vi "{TMPL} MAIN - App.vi"() -> ()   [LabVIEW 2018, in "TLB` Template.lvlib" / "{TMPL} TLB`.lvclass"]
uses:
  {TMPL} TLB`.lvclass
  Application Components/Trigger API/System Trigger.ctl
  State Machine/State.ctl
  Core Components/Error Handler/TLB` Error Handler.lvclass
  Application Components/Configuration/{TMPL} Station Configuration.lvclass
  {TMPL} TLB`.lvclass/{TMPL} TLB`.ctl
  <vilib>/Utility/error.llb/Error Cluster From Error Code.vi
  <vilib>/ErrorRing/Error Ring.xnode
  Application Components/Trigger API/{TMPL} Trigger API.lvlib
  TLB` Template.lvlib
  Core Components/Actions/Actions.lvlib
  Core Components/Dependencies/TLB`_Dependencies.lvlib
panel:
  in  "Active Tab Selector":i32(listbox)
  in  "Connect Instrument":bool
  in  "Disconnect Instrument":bool
  in  "Initiate Analysis":bool
  in  "Stop Analysis":bool
  in  "Load Configuration":bool
  in  "Save Configuration":bool
  in  "Exit":bool
  in  "Main Tab":T1(tab)
  in  "VISA":refnum<visa-resource-name>
  out "error out":errorcluster
  in  "Preferences Button":bool
  out "Waveform Graph - Light":dbl[](graph)
  out "State":string
  out "Status":string
  # "TLB` Measurement Template"
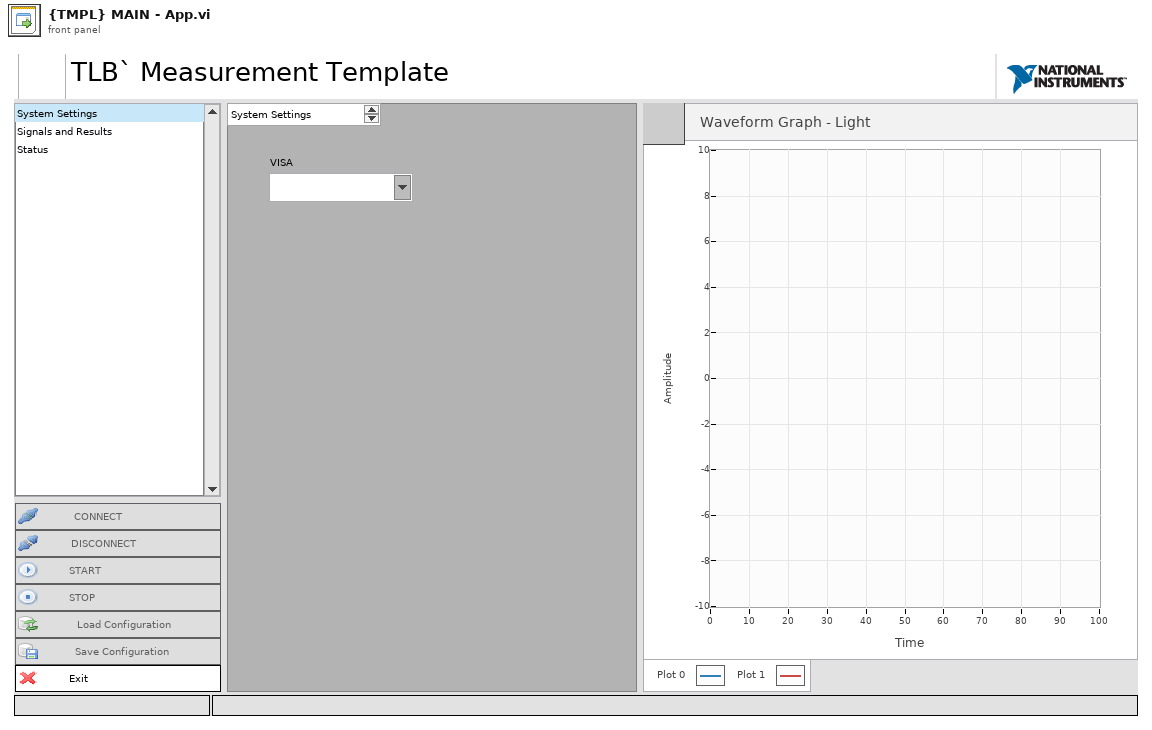
[diagram p1: front panel]
types:
  T1 = enum32{"System Settings", "Signals and Results", "Status"}
  T2 = typedef "TLB` Template.lvlib/{TMPL} TLB`.lvclass/State.ctl" = enum16{"<Startup>", "Idle", "Connected", "Monitoring", "Sweeping", "<Shutdown>", "<Error>"}
  T3 = enum16{"Close Display", "Clear References", "Close Error Handler"}
  T4 = enum16{"Clear SR", "Set Display", "Set Shifter", "Initialize Events", "Init Q"}
  T5 = typedef "TLB` Template.lvlib/{TMPL} Trigger API.lvlib/System Trigger.ctl" = enum16{"<None>", "Connect", "Start Acquisition", "Stop Acquisition", "Disconnect", "Load Configuration", "Save Configuration", "<Return to Safe State Actions>", "<Cache User Parameters>", "<Close Application>", "<Error>"}
  T6 = refnum<class "{TMPL} Station Configuration.lvclass">
  T7 = typedef "TLB` Template.lvlib/_UI CORE Event References.ctl" = cluster{"Exit Event":refnum<user-event>, "State Indicator":refnum<user-event>, "Status Indicator":refnum<user-event>}
  T8 = typedef "TLB` Template.lvlib/_UI APP Event References.ctl" = cluster{"Exit Event":refnum<user-event>}
  T9 = enum32{"Invalid", "Standard", "Closed", "Hidden", "Minimized", "Maximized"}
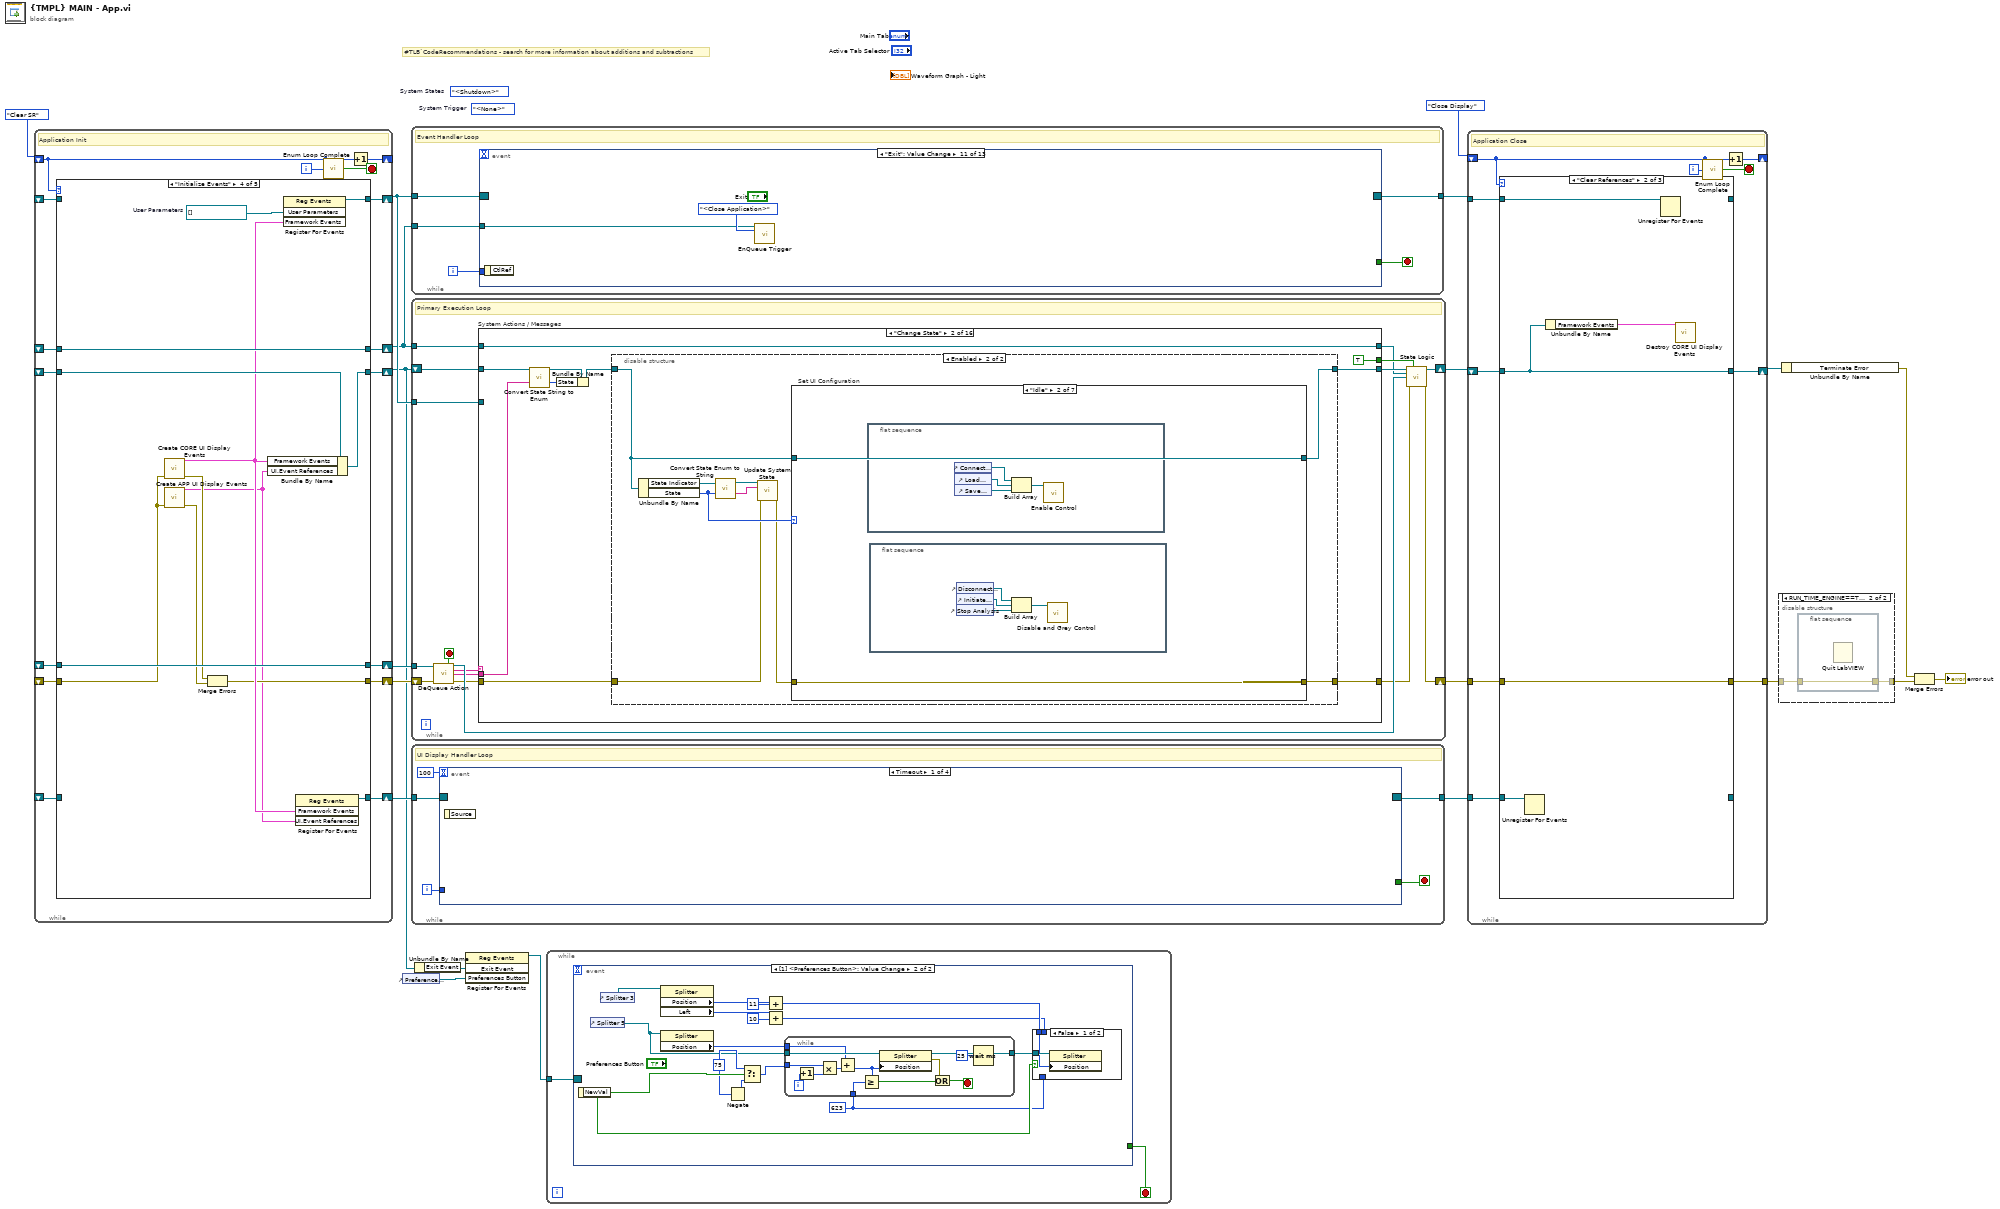
[diagram p0: block diagram]
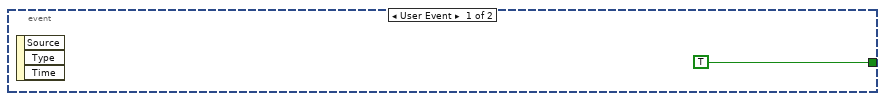
[diagram p2: hidden frame]
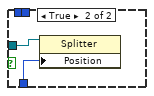
[diagram p3: hidden frame]
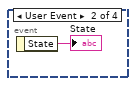
[diagram p4: hidden frame]
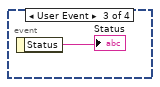
[diagram p5: hidden frame]
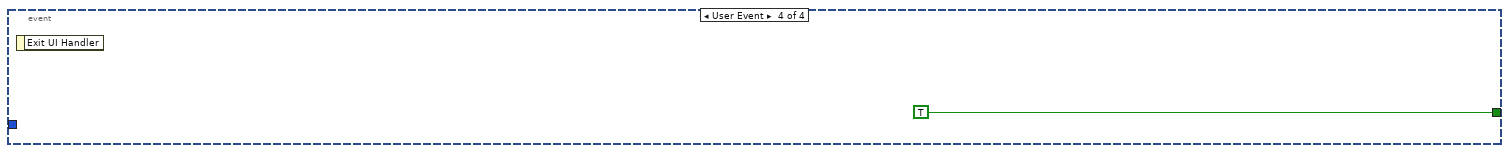
[diagram p6: hidden frame]
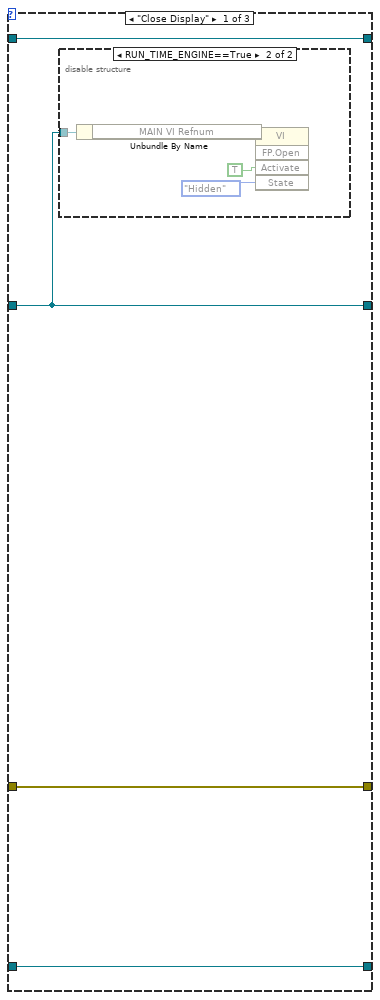
[diagram p8: hidden frame]
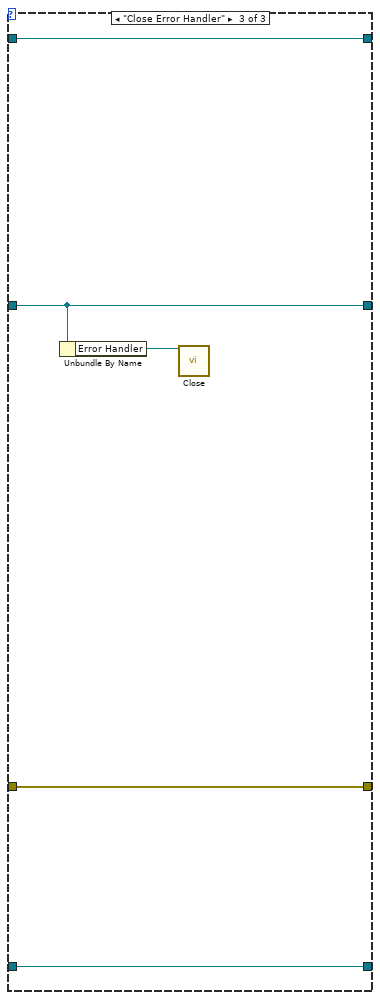
[diagram p10: hidden frame]
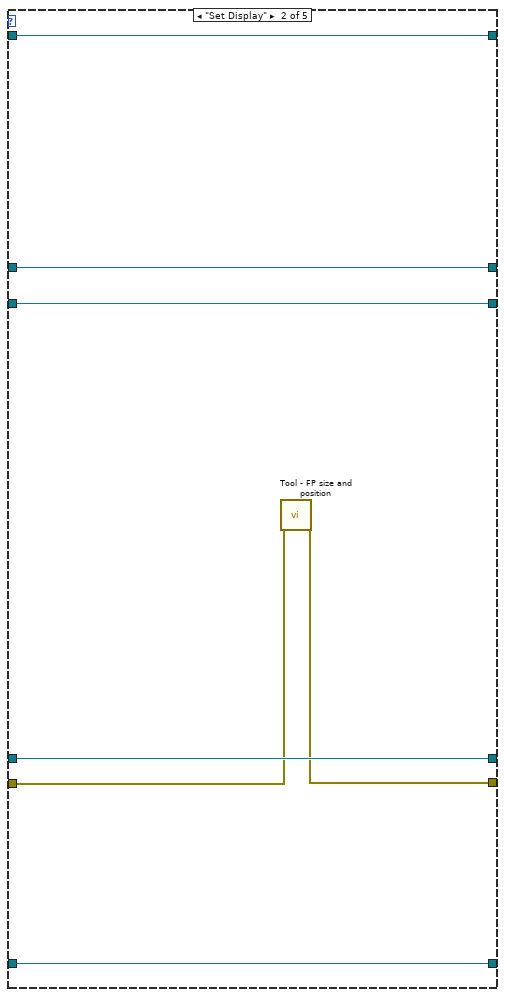
[diagram p12: hidden frame]
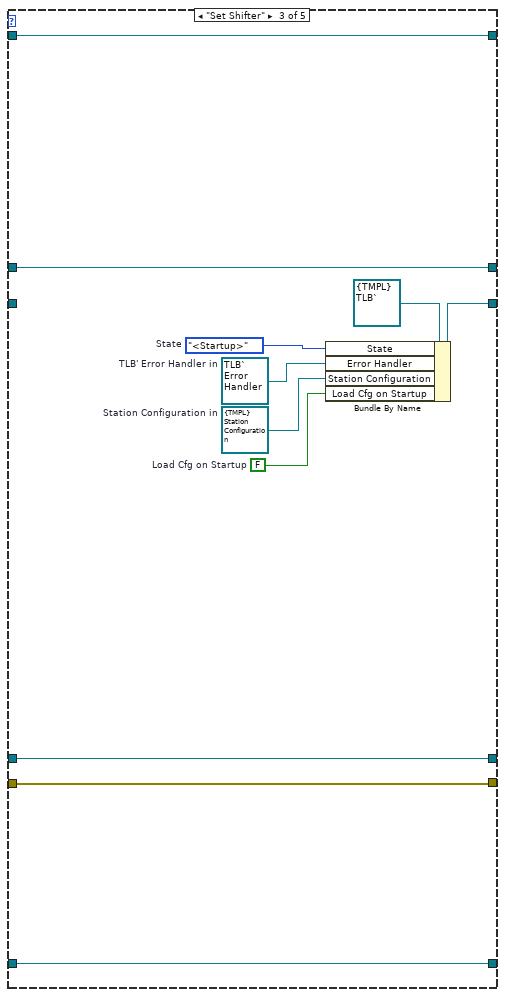
[diagram p13: hidden frame]
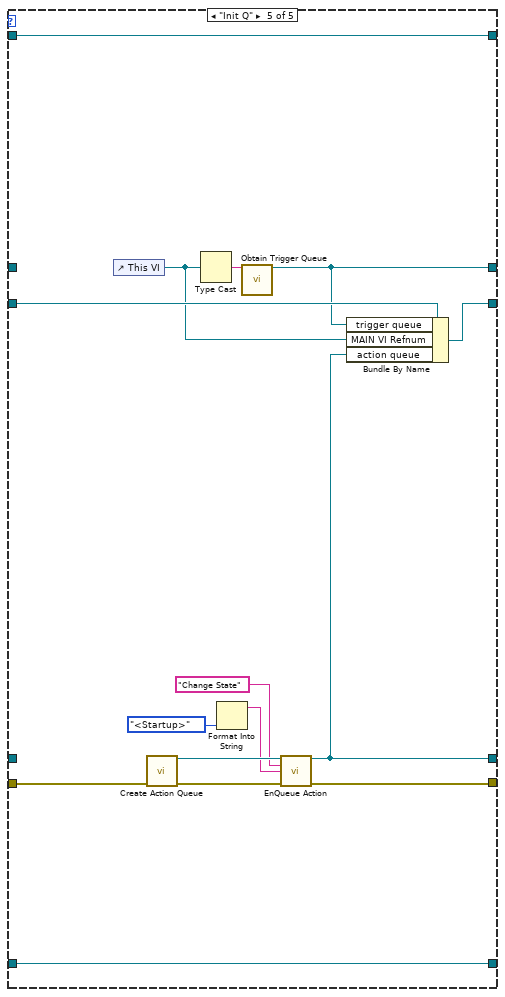
[diagram p14: hidden frame]
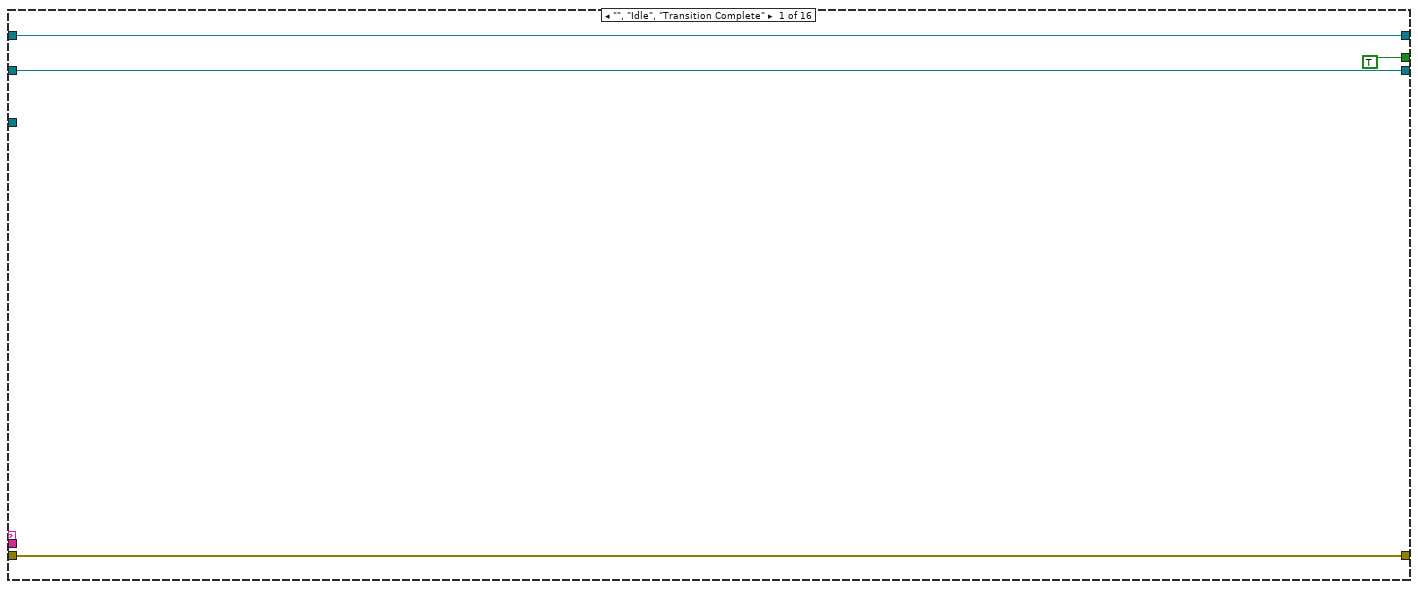
[diagram p15: hidden frame]
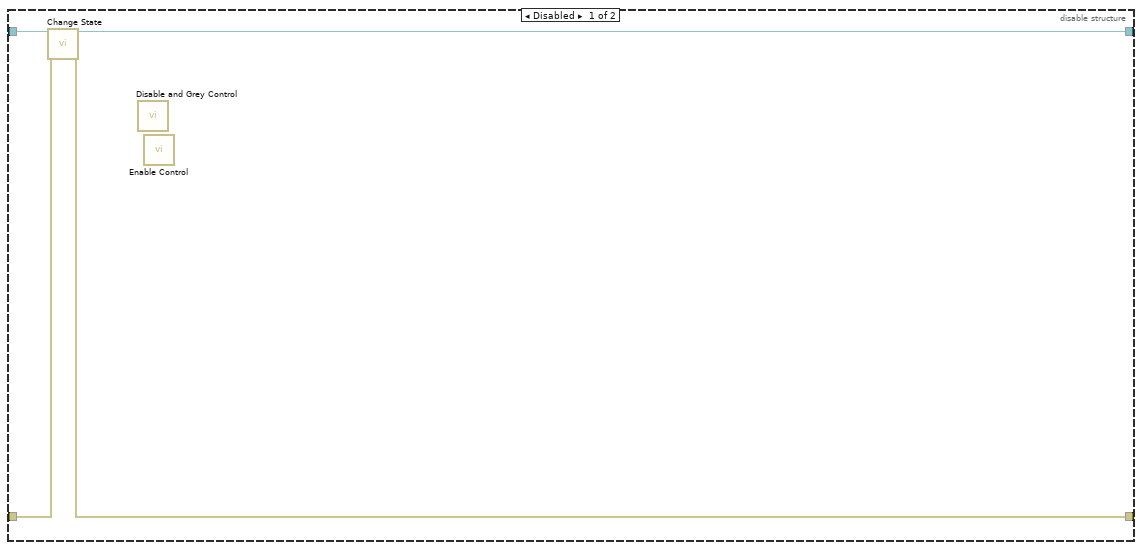
[diagram p16: hidden frame]
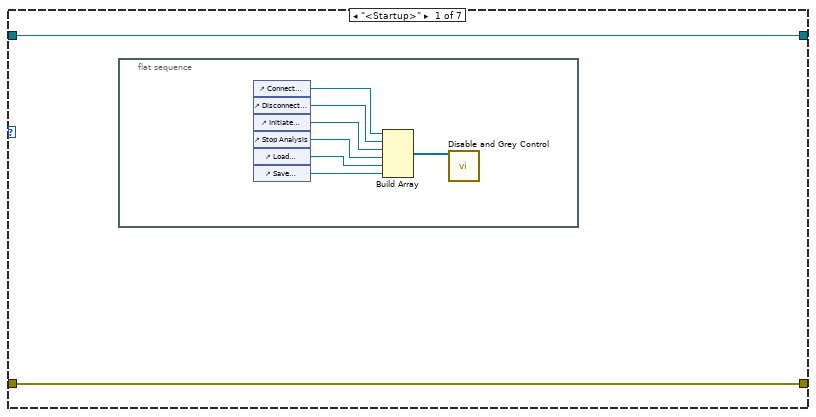
[diagram p17: hidden frame]
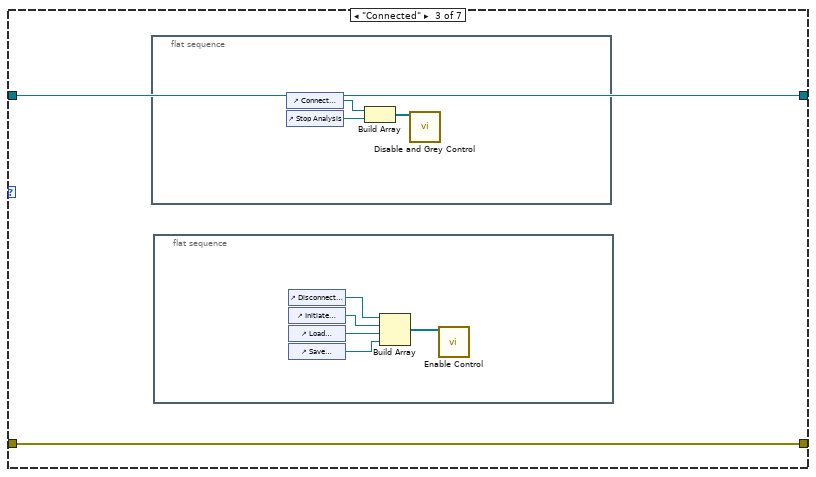
[diagram p18: hidden frame]
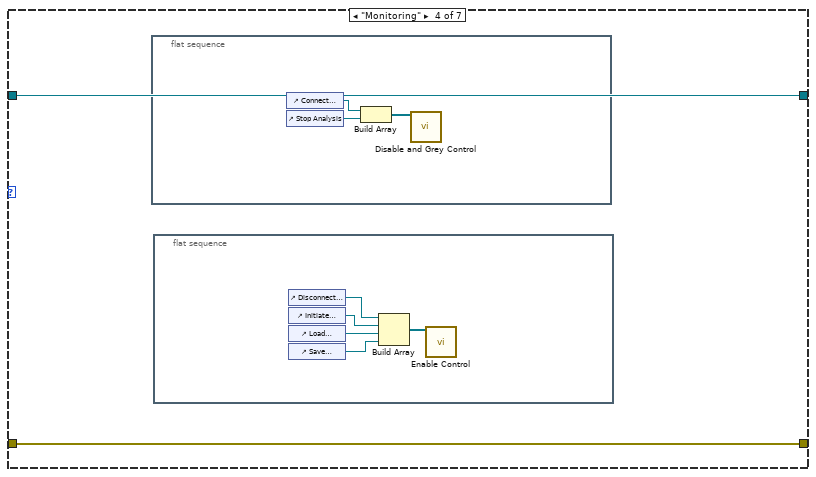
[diagram p19: hidden frame]
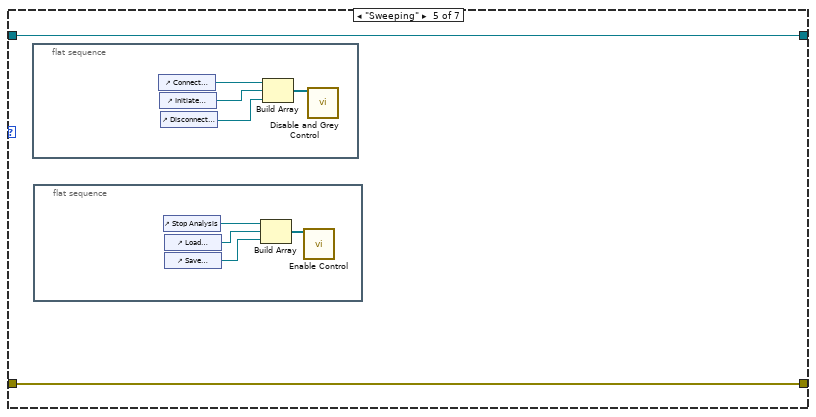
[diagram p20: hidden frame]
diagram:
  (unwired) State."<Shutdown>"  # System States
  (unwired) System_Trigger."<None>"  # System Trigger
  # "#TLB`CodeRecommendations - search for more information about additions and subtractions"
  n1 = while {
    shift-right: [w32] -> _
    shift-left: T4."Clear SR" -> [w21]
    shift-right: [w36] -> w20
    shift-left: _ -> [w31]
    shift-right: [w33] -> w15
    shift-left: _ -> [w30]
    shift-right: [w35] -> w14
    shift-left: _ -> [w29]
    shift-right: [w34] -> w4
    shift-left: _ -> [w28]
    shift-right: [w27] -> w10
    shift-left: _ -> [w26]
    shift-right: [w25] -> w13
    shift-left: _ -> [w24]
    i -> [w22]
    stop <- w23 stop-if-true
    # "Application Init"
    n2 = case shown="\"Initialize Events\"" w21 {
      tunnel: [_ w41 w54 w67 w68] -> w36
      tunnel: [_ w39 w53 w57 w74] -> w33
      tunnel: [_ w43 w49 w65 w80] -> w34
      tunnel: [_ w42 w52 w64 w82] -> w35
      tunnel: w31 -> [_ w41 w54 w67 _]
      tunnel: w30 -> [_ w40 w53 w56 w76]
      tunnel: w29 -> [_ w42 w52 _ w82]
      tunnel: w28 -> [_ w43 _ w66 w81]
      tunnel: [_ w38 w51 w63 w69] -> w27
      tunnel: w26 -> [_ w38 w51 w63 _]
      tunnel: [_ w37 w47 w61 w77] -> w25
      tunnel: w24 -> [_ w37 w47 _ w77]
      frame "Clear SR" {
      }
      frame "Set Display" {
        n3 = call "Tool - FP size and position.vi"("error in (no error)"=w40) -> ("error out"=w39:errorcluster)  [unwired: 17 in, 1 out]
      }
      frame "Set Shifter" {
        w44 = FALSE  # Load Cfg on Startup
        w45 = T6 refnum  # Station Configuration in
        w46 = refnum<class "TLB` Error Handler.lvclass"> refnum  # TLB' Error Handler in
        w50 = State."<Startup>"  # State
        n4 = Bundle By Name(cluster=refnum<class "{TMPL} TLB`.lvclass"> refnum ("TLB` Template.lvlib:TLB' Template.lvclass"), "State"=w50, "Error Handler"=w46, "Station Configuration"=w45, "Load Cfg on Startup"=w44) -> (w49:refnum<class "{TMPL} TLB`.lvclass">)
      }
      frame "Initialize Events" {
        w62 = refnum<vi>[] []  # User Parameters
        n5 = call "Create CORE UI Display Events.vi"("error in"=w56) -> ("Framework Events"=w60:T7, "error out"=w59:errorcluster)  [unwired: 13 in]
        n6 = call "Create APP UI Display Events.vi"("error in"=w56) -> ("UI.Event References"=w55:T8, "error out"=w58:errorcluster)  [unwired: 13 in]
        n7 = Merge Errors(w59, w58) -> (w57:errorcluster)
        n8 = Bundle By Name(cluster=w66, "Framework Events"=w60, "UI.Event References"=w55) -> (w65:refnum<class "{TMPL} TLB`.lvclass">)
        n9 = register-events(w62, w60) -> (reference out=w64:refnum<event-registration>)  [unwired: 2 in, 1 out]
        n10 = register-events(w60, w55) -> (reference out=w61:refnum<event-registration>)  [unwired: 2 in, 1 out]
      }
      frame "Init Q" {
        n11 = control-ref of="This VI"() -> (w79:refnum<vi>)
        n12 = call "Create Action Queue.vi"("error in"=w76) -> ("action queue out"=w73:refnum<queue>, "error out"=w75:errorcluster)  [unwired: 13 in]
        n13 = Type Cast(x=w79) -> (*(type *) &x=w70:string)  [unwired: 1 in]
        n14 = Format Into String(State."<Startup>" ("State")) -> (resulting string=w71:string)  [unwired: 3 in, 1 out]
        n15 = call "Obtain Trigger Queue.vi"("trigger queue name"=w70) -> ("trigger queue out"=w69:refnum<queue>)  [unwired: 13 in, 1 out]
        n16 = call "EnQueue Action.vi"("action queue in"=w73, "action"="Change State" ("Message Name"), "data in"=w71, "error in"=w75) -> ("action queue out"=w68:refnum<queue>, "error out"=w74:errorcluster)  [unwired: 10 in]
        n17 = Bundle By Name(cluster=w81, "trigger queue"=w69, "MAIN VI Refnum"=w79, "action queue"=w68) -> (w80:refnum<class "{TMPL} TLB`.lvclass">)
      }
    }
    n18 = call "Enum Loop Complete.vi"("Current State Enum"=w21, "Itteration"=w22) -> ("Loop Complete?"=w23:bool)  [unwired: 12 in, 1 out]
    n19 = Increment(x=w21) -> (x+1=w32:T4)
  }
  n20 = control-ref of="Preferences Button"() -> (w1:refnum<vi>)
  n21 = while {
    shift-right: [w93] -> w12
    shift-left: w15 -> [w88]
    shift-right: [w95] -> w16
    shift-left: w4 -> [w97]
    tunnel: w20 -> [w89]
    tunnel: w14 -> [w96]
    tunnel: w10 -> [w92]
    stop <- w87 stop-if-true
    # "Primary Execution Loop"
    n22 = call "DeQueue Action.vi"("action queue in"=w89, "error in"=w88) -> ("exit?"=w87:bool, "action queue out"=w98:refnum<queue>, "action"=w85:string, "action value"=w83:string, "error out"=w86:errorcluster)  [unwired: 8 in, 1 out]
    n23 = case "System Actions / Messages" shown="\"Change State\"" w85 {
      selector: w85 -> [_ _ _ _ _ _ _ _ _ _ _ _ _ _ _ w275]
      tunnel: [w102 w109 w190 w194 w195 w204 w213 w229 w238 w244 w247 w252 w257 w258 w270 w274] -> w90
      tunnel: w86 -> [w102 w108 w190 w194 w195 w207 w213 w229 w236 w244 w247 w251 w257 w259 w271 _]
      tunnel: w97 -> [w99 w107 w187 w193 w198 w205 w216 w228 w232 w243 w246 w254 w256 w262 w273 w277]
      tunnel: [w99 w103 w191 w193 w197 w210 w219 w228 w233 w243 w246 w254 w256 w261 w272 w277] -> w94
      tunnel: w96 -> [_ _ _ _ _ _ w217 _ _ _ _ _ _ _ _ _]
      tunnel: [w100 w110 w189 w192 w199 w211 w218 w227 w241 w242 w245 w249 w255 w265 w266 w276] -> w84
      tunnel: w92 -> [w100 w110 w189 w192 w199 w211 w218 w227 w241 w242 w245 w249 w255 w265 w266 w276]
      tunnel: [TRUE TRUE _ _ _ _ _ _ _ _ _ _ _ _ _ _] -> w91
      tunnel: w83 -> [_ w106 _ _ _ _ _ _ _ _ _ _ _ _ _ _]
      frame "", "Idle", "Transition Complete" {
      }
      frame "Change State" {
        n24 = call "Convert State String to Enum.vi"("state in"=w106) -> ("state out"=w105:T2)  [unwired: 13 in, 1 out]
        n25 = Bundle By Name(cluster=w107, "State"=w105) -> (w104:refnum<class "{TMPL} TLB`.lvclass">)
        n26 = disable-structure shown="Enabled" {
          disable-tunnel: [w115 w116] -> w109
          disable-tunnel: w108 -> [w114 w117]
          disable-tunnel: w104 -> [w113 w119]
          disable-tunnel: [w112 w118] -> w103
          frame Disabled {
            n27 = call "Change State.vi"("TLB' data in"=w113, "error in"=w114) -> ("TLB' data out"=w112:refnum<class "{TMPL} TLB`.lvclass">, "error out"=w115:errorcluster)  [unwired: 12 in]
            n28 = call "Disable and Grey Control.vi"() -> ()  [unwired: 15 in, 1 out]
            n29 = call "Enable Control.vi"() -> ()  [unwired: 15 in, 1 out]
          }
          frame Enabled {
            n30 = Unbundle By Name(w119) -> ("State Indicator"=w120:refnum<user-event>, "State"=w123:T2)
            n31 = call "Convert State Enum to String.vi"("state in"=w123) -> ("state out"=w121:string)  [unwired: 13 in, 1 out]
            n32 = call "Update System State.vi"("State Indicator"=w120, "system state message"=w121, "error in"=w117) -> ("error out"=w122:errorcluster)  [unwired: 12 in]
            n33 = case "Set UI Configuration" shown="\"Idle\"" w123 {
              tunnel: [w124 w134 w144 w154 w164 w176 w184] -> w116
              tunnel: w122 -> [w124 w134 w144 w154 w164 w176 w184]
              tunnel: [w125 w133 w143 w153 w163 w175 w185] -> w118
              tunnel: w119 -> [w125 w133 w143 w153 w163 w175 w185]
              frame "<Startup>" {
                n34 = flat-sequence {
                  frame #0 {
                    n35 = control-ref of="Connect Instrument"() -> (w132:refnum<vi>)
                    n36 = control-ref of="Disconnect Instrument"() -> (w131:refnum<vi>)
                    n37 = control-ref of="Initiate Analysis"() -> (w130:refnum<vi>)
                    n38 = control-ref of="Stop Analysis"() -> (w129:refnum<vi>)
                    n39 = control-ref of="Load Configuration"() -> (w128:refnum<vi>)
                    n40 = control-ref of="Save Configuration"() -> (w127:refnum<vi>)
                    n41 = Build Array(w132, w131, w130, w129, w128, w127) -> (w126:refnum<vi>[])
                    n42 = call "Disable and Grey Control.vi"("Control Ref"=w126) -> ()  [unwired: 14 in, 1 out]
                  }
                }
              }
              frame "Idle" {
                n43 = flat-sequence {
                  frame #0 {
                    n44 = control-ref of="Connect Instrument"() -> (w140:refnum<vi>)
                    n45 = control-ref of="Load Configuration"() -> (w142:refnum<vi>)
                    n46 = control-ref of="Save Configuration"() -> (w141:refnum<vi>)
                    n47 = Build Array(w140, w142, w141) -> (w139:refnum<vi>[])
                    n48 = call "Enable Control.vi"("Control Ref"=w139) -> ()  [unwired: 14 in, 1 out]
                  }
                }
                n49 = flat-sequence {
                  frame #0 {
                    n50 = control-ref of="Disconnect Instrument"() -> (w138:refnum<vi>)
                    n51 = control-ref of="Initiate Analysis"() -> (w137:refnum<vi>)
                    n52 = control-ref of="Stop Analysis"() -> (w136:refnum<vi>)
                    n53 = Build Array(w138, w137, w136) -> (w135:refnum<vi>[])
                    n54 = call "Disable and Grey Control.vi"("Control Ref"=w135) -> ()  [unwired: 14 in, 1 out]
                  }
                }
              }
              frame "Connected" {
                n55 = flat-sequence {
                  frame #0 {
                    n56 = control-ref of="Connect Instrument"() -> (w152:refnum<vi>)
                    n57 = control-ref of="Stop Analysis"() -> (w151:refnum<vi>)
                    n58 = Build Array(w152, w151) -> (w150:refnum<vi>[])
                    n59 = call "Disable and Grey Control.vi"("Control Ref"=w150) -> ()  [unwired: 14 in, 1 out]
                  }
                }
                n60 = flat-sequence {
                  frame #0 {
                    n61 = control-ref of="Disconnect Instrument"() -> (w149:refnum<vi>)
                    n62 = control-ref of="Initiate Analysis"() -> (w148:refnum<vi>)
                    n63 = control-ref of="Load Configuration"() -> (w147:refnum<vi>)
                    n64 = control-ref of="Save Configuration"() -> (w146:refnum<vi>)
                    n65 = Build Array(w149, w148, w147, w146) -> (w145:refnum<vi>[])
                    n66 = call "Enable Control.vi"("Control Ref"=w145) -> ()  [unwired: 14 in, 1 out]
                  }
                }
              }
              frame "Monitoring" {
                n67 = flat-sequence {
                  frame #0 {
                    n68 = control-ref of="Connect Instrument"() -> (w162:refnum<vi>)
                    n69 = control-ref of="Stop Analysis"() -> (w161:refnum<vi>)
                    n70 = Build Array(w162, w161) -> (w160:refnum<vi>[])
                    n71 = call "Disable and Grey Control.vi"("Control Ref"=w160) -> ()  [unwired: 14 in, 1 out]
                  }
                }
                n72 = flat-sequence {
                  frame #0 {
                    n73 = control-ref of="Disconnect Instrument"() -> (w159:refnum<vi>)
                    n74 = control-ref of="Initiate Analysis"() -> (w158:refnum<vi>)
                    n75 = control-ref of="Load Configuration"() -> (w157:refnum<vi>)
                    n76 = control-ref of="Save Configuration"() -> (w156:refnum<vi>)
                    n77 = Build Array(w159, w158, w157, w156) -> (w155:refnum<vi>[])
                    n78 = call "Enable Control.vi"("Control Ref"=w155) -> ()  [unwired: 14 in, 1 out]
                  }
                }
              }
              frame "Sweeping" {
                n79 = flat-sequence {
                  frame #0 {
                    n80 = control-ref of="Connect Instrument"() -> (w172:refnum<vi>)
                    n81 = control-ref of="Initiate Analysis"() -> (w170:refnum<vi>)
                    n82 = control-ref of="Disconnect Instrument"() -> (w169:refnum<vi>)
                    n83 = Build Array(w172, w170, w169) -> (w171:refnum<vi>[])
                    n84 = call "Disable and Grey Control.vi"("Control Ref"=w171) -> ()  [unwired: 14 in, 1 out]
                  }
                }
                n85 = flat-sequence {
                  frame #0 {
                    n86 = control-ref of="Stop Analysis"() -> (w166:refnum<vi>)
                    n87 = control-ref of="Load Configuration"() -> (w168:refnum<vi>)
                    n88 = control-ref of="Save Configuration"() -> (w167:refnum<vi>)
                    n89 = Build Array(w166, w168, w167) -> (w165:refnum<vi>[])
                    n90 = call "Enable Control.vi"("Control Ref"=w165) -> ()  [unwired: 14 in, 1 out]
                  }
                }
              }
              frame "<Shutdown>" {
                n91 = flat-sequence {
                  frame #0 {
                    n92 = control-ref of="Connect Instrument"() -> (w183:refnum<vi>)
                    n93 = control-ref of="Disconnect Instrument"() -> (w182:refnum<vi>)
                    n94 = control-ref of="Initiate Analysis"() -> (w181:refnum<vi>)
                    n95 = control-ref of="Stop Analysis"() -> (w180:refnum<vi>)
                    n96 = control-ref of="Load Configuration"() -> (w179:refnum<vi>)
                    n97 = control-ref of="Save Configuration"() -> (w178:refnum<vi>)
                    n98 = Build Array(w183, w182, w181, w180, w179, w178) -> (w177:refnum<vi>[])
                    n99 = call "Disable and Grey Control.vi"("Control Ref"=w177) -> ()  [unwired: 14 in, 1 out]
                  }
                }
                n100 = control-ref of="Preferences Button"() -> (w174:refnum<vi>)
                n101 = property class="Bool (strict)"(reference=w174, "Val(Sgnl)"=TRUE ("Value (Signaling)")) -> ()  [unwired: 1 in, 2 out]
              }
              frame "<Error>" {
              }
            }
          }
        }
      }
      frame "Cache User Parameters" {
        n102 = Bundle By Name(cluster=w187, "Active Item Tag"="" ("User Data.Active Item Tag"), "VISA"="VISA") -> (w191:refnum<class "{TMPL} TLB`.lvclass">)
      }
      frame "/*********INITialize********/" {
      }
      frame "INIT::Load Application Base Path" {
        n103 = disable-structure shown="Default" {
          disable-tunnel: [w200 w202] -> w196
          frame condition #0 (active) {
            n104 = Current VI's Path() -> (path=w201:path)
            n105 = Strip Path(path=w201) -> (stripped path=w200:path)  [unwired: 1 out]
          }
          frame condition #1 {
            n106 = call <vilib>:"Application Directory.vi"() -> ("Application Directory"=w202:path)
          }
        }
        n107 = Bundle By Name(cluster=w198, "Application Base Path"=w196) -> (w197:refnum<class "{TMPL} TLB`.lvclass">)
      }
      frame "INIT::Initialize Error Handler" {
        n108 = Unbundle By Name(w205) -> ("Application Base Path"=w212:path)
        n109 = Unbundle By Name(w205) -> ("Error Handler"=w206:refnum<class "TLB` Error Handler.lvclass">)
        n110 = Build Path(base path=w212, name or relative path="System Level Errors\\System Errors.txt") -> (appended path=w208:path)
        n111 = call-dynamic "Open.vi"("error handler in"=w206, "error log path in"=w208, "error in"=w207) -> ("error handler out"=w209:refnum<class "TLB` Error Handler.lvclass">, "error out"=w204:errorcluster)  [unwired: 11 in]
        n112 = Bundle By Name(cluster=w205, "Error Handler"=w209) -> (w210:refnum<class "{TMPL} TLB`.lvclass">)
      }
      frame "INIT::Register User Parameters" {
        n113 = disable-structure shown="Enabled" {
          disable-tunnel: [w220 refnum<vi>[] [] ("User Parameter Controls")] -> w215
          frame Enabled {
            n114 = stacked-sequence "Stacked Sequence Structure :: Allows for a lot of controls" {
              tunnel: [w222] -> w220
              frame #0 {
                n115 = control-ref of="VISA"() -> (w221:refnum<vi>)
                n116 = Build Array(w221) -> (w222:refnum<vi>[])
              }
            }
          }
          frame Disabled {
          }
        }
        n117 = Build Array (concatenate)(w215) -> (w214:refnum<vi>[])
        n118 = register-events(reference=w217, w214) -> ()  [unwired: 2 in, 2 out]
        n119 = Bundle By Name(cluster=w216, "User Parameter Controls"=w214) -> (w219:refnum<class "{TMPL} TLB`.lvclass">)
      }
      frame "INIT::FP Values" {
        w224 = 0
        # "#TLB`CodeRecommendations - initialize FP values here"
        n120 = property on="Main Tab" class="TabCtl (strict)"() -> ("Pages"=w226:refnum<vi>[])  [unwired: 2 in, 2 out]
        n121 = for {
          tunnel: w226 -> [w231] mode=indexing
          tunnel: [w230] -> w225 mode=indexing
          n122 = property class="Page"(reference=w231) -> ("TabCaption"=w230:string)  [unwired: 1 in, 2 out]
        }
        n123 = local write "Active Tab Selector"(w224) -> ()
        n124 = local write "Main Tab"(w224) -> ()
        n125 = property on="Active Tab Selector" class="LstBox (strict)"("Item Names"=w225) -> ()  [unwired: 2 in, 2 out]
      }
      frame "CFG::Load Station Configuration" {
        n126 = Unbundle By Name(w232) -> ("Application Base Path"=w240:path)
        n127 = Unbundle By Name(w232) -> ("Station Configuration"=w235:T6)
        n128 = Build Path(base path=w240, name or relative path="System Configuration\\Station Configuration.ini") -> (appended path=w237:path)
        n129 = call-dynamic "Load Configuration.vi"("INI Station Configuration in"=w235, "INI file path in"=w237, "error in"=w236) -> ("INI Station Configuration out"=w234:T6, "error out"=w238:errorcluster)  [unwired: 11 in]
        n130 = Bundle By Name(cluster=w232, "Station Configuration"=w234) -> (w233:refnum<class "{TMPL} TLB`.lvclass">)
      }
      frame "/*********PRImary EXEcution********/" {
      }
      frame "/*********SHUTDOWN********/" {
      }
      frame "Exit" {
        w250 = refnum<class> refnum  # event data
        # "Don't wire 'Error In'\nMust Execute Regardless"
        n131 = Unbundle By Name(w254) -> ("Exit Event"=w248:refnum<user-event>)
        n132 = Generate User Event(user event=w248, event data cluster=w250) -> (error out=w253:errorcluster)  [unwired: 2 in, 1 out]
        n133 = Merge Errors(w251, w253) -> (w252:errorcluster)
      }
      frame "/*********ERRor Handler********/" {
      }
      frame "ERR::Log" {
        n134 = Unbundle By Name(w262) -> ("Error Handler"=w264:refnum<class "TLB` Error Handler.lvclass">)
        n135 = call-dynamic "Log.vi"("error handler in"=w264) -> ("error handler out"=w263:refnum<class "TLB` Error Handler.lvclass">, "error out"=w260:errorcluster)  [unwired: 13 in]
        n136 = Bundle By Name(cluster=w262, "Error Handler"=w263) -> (w261:refnum<class "{TMPL} TLB`.lvclass">)
        n137 = Merge Errors(w259, w260) -> (w258:errorcluster)
      }
      frame "ERR::Dialog" {
        n138 = Unbundle By Name(w273) -> ("Error Handler"=w269:refnum<class "TLB` Error Handler.lvclass">)
        n139 = call-dynamic "Dialog.vi"("error handler in"=w269, "trigger queue in"=w266) -> ("error handler out"=w268:refnum<class "TLB` Error Handler.lvclass">, "error out"=w267:errorcluster)  [unwired: 12 in]
        n140 = Merge Errors(w271, w267) -> (w270:errorcluster)
        n141 = Bundle By Name(cluster=w273, "Error Handler"=w268) -> (w272:refnum<class "{TMPL} TLB`.lvclass">)
      }
      frame Default {
        n142 = xnode "Error Ring"("parameter 0"=w275) -> ("error out"=w274:errorcluster)
      }
    }
    n143 = call "State Logic.vi"("TLB' data in"=w94, "process state logic enable"=w91, "trigger queue in"=w84, "action queue in"=w98, "error in"=w90) -> ("TLB' data out"=w95:refnum<class "{TMPL} TLB`.lvclass">, "error out"=w93:errorcluster)  [unwired: 9 in]
  }
  n144 = while {
    tunnel: w13 -> [w289]
    tunnel: [w285] -> w11
    i -> [w288]
    stop <- w287 stop-if-true
    # "UI Display Handler Loop"
    n145 = event shown="[0] Timeout" {
      selector: w289 -> [_ _ _ _]
      dyn-events: [_ _ _ _] -> w285
      timeout: 100 -> [_ _ _ _]
      tunnel: w288 -> [_ _ _ _]
      tunnel: [_ _ _ TRUE] -> w287
      event Timeout {
        n146 = event-data() -> ()  [unwired: 2 out]
      }
      event User Event {
        n147 = event-data() -> ("State"=→"State":string)  [unwired: 1 out]
      }
      event User Event {
        n148 = event-data() -> ("Status"=→"Status":string)  [unwired: 1 out]
      }
      event User Event {
        n149 = event-data() -> ()  [unwired: 2 out]
      }
    }
  }
  n150 = while {
    tunnel: w14 -> [w296]
    tunnel: [w295] -> w17
    tunnel: w10 -> [w293]
    i -> [w294]
    stop <- w297 stop-if-true
    # "Event Handler Loop"
    n151 = event shown="[10] \"Exit\": Value Change" {
      selector: w296 -> [_ _ _ _ _ _ _ _ _ _ _ _ _]
      dyn-events: [_ _ _ _ _ _ _ _ _ _ _ _ _] -> w295
      timeout: _ -> [_ _ _ _ _ _ _ _ _ _ _ _ _]
      tunnel: [_ _ TRUE ("NewVal") _ _ _ _ _ _ _ _ _ _] -> w297
      tunnel: w294 -> [_ _ _ _ _ _ _ _ _ _ _ _ _]
      tunnel: w293 -> [w298 _ w310 w314 w317 w319 w321 w323 w325 w327 w328 _ _]
      event Panel Close? {
        w300 = TRUE  # Discard?
        n152 = event-data() -> ()  [unwired: 2 out]
        n153 = call "EnQueue Trigger.vi"("trigger queue in"=w298, "system trigger"=System_Trigger."<Close Application>" ("System Trigger")) -> ()  [unwired: 12 in, 2 out]
        n154 = event-data("Discard?"=w300) -> ()  [unwired: 1 in, 1 out]
      }
      event Mouse Down {
        n155 = event-data() -> ("Button"=w301:u16, "Mods.Double Click"=w302:bool)  [unwired: 1 out]
        n156 = Equal?(x=u16 2, y=w301) -> (x = y?=w304:bool)
        n157 = Compound Arithmetic op=AND(w304, w302) -> (w303:bool)
        n158 = case "Toggle Menu Visibility :: double RIGHT click on logo" shown="True" w303 {
          frame False {
          }
          frame True {
            n159 = property class="VI"() -> (reference out=w308:refnum<vi>, "TB.Visible"=w307:bool)  [unwired: 2 in, 1 out]
            n160 = Not(x=w307) -> (.not. x?=w306:bool)
            n161 = property class="VI"(reference=w308, "TB.Visible"=w306, "Front Panel.ShowMenuBar"=w306) -> ()  [unwired: 1 in, 2 out]
          }
        }
      }
      event User Event {
        n162 = event-data() -> ()  [unwired: 2 out]
        n163 = call "EnQueue Trigger.vi"("trigger queue in"=w310, "system trigger"=System_Trigger."<Close Application>" ("System Trigger")) -> ()  [unwired: 12 in, 2 out]
      }
      event Value Change {
        n164 = event-data() -> ()  [unwired: 2 out]
        n165 = call "EnQueue Trigger.vi"("trigger queue in"=w314, "system trigger"=System_Trigger."<Cache User Parameters>" ("System Trigger")) -> ("trigger queue out"=w313:refnum<queue>)  [unwired: 12 in, 1 out]
        n166 = event "use this event case to register a SPEICIFIC 'User Parameter' for a SPECIFIC action" shown="[0] Timeout" {
          selector: _ -> [_]
          dyn-events: _ -> [_]
          timeout: 0 -> [_]
          tunnel: w313 -> [_]
          event Timeout {
            n167 = event-data() -> ()  [unwired: 1 in, 1 out]
          }
        }
      }
      event "Connect Instrument": Value Change {
        n168 = event-data() -> ()  [unwired: 2 out]
        n169 = call "EnQueue Trigger.vi"("trigger queue in"=w317, "system trigger"=System_Trigger."Connect" ("System Trigger")) -> ()  [unwired: 12 in, 2 out]
      }
      event "Disconnect Instrument": Value Change {
        n170 = event-data() -> ()  [unwired: 2 out]
        n171 = call "EnQueue Trigger.vi"("trigger queue in"=w319, "system trigger"=System_Trigger."Disconnect" ("System Trigger")) -> ()  [unwired: 12 in, 2 out]
      }
      event "Initiate Analysis": Value Change {
        n172 = event-data() -> ()  [unwired: 2 out]
        n173 = call "EnQueue Trigger.vi"("trigger queue in"=w321, "system trigger"=System_Trigger."Start Acquisition" ("System Trigger")) -> ()  [unwired: 12 in, 2 out]
      }
      event "Stop Analysis": Value Change {
        n174 = event-data() -> ()  [unwired: 2 out]
        n175 = call "EnQueue Trigger.vi"("trigger queue in"=w323, "system trigger"=System_Trigger."Stop Acquisition" ("System Trigger")) -> ()  [unwired: 12 in, 2 out]
      }
      event "Save Configuration": Value Change {
        n176 = event-data() -> ()  [unwired: 2 out]
        n177 = call "EnQueue Trigger.vi"("trigger queue in"=w325, "system trigger"=System_Trigger."Save Configuration" ("System Trigger")) -> ()  [unwired: 12 in, 2 out]
      }
      event "Load Configuration": Value Change {
        n178 = event-data() -> ()  [unwired: 2 out]
        n179 = call "EnQueue Trigger.vi"("trigger queue in"=w327, "system trigger"=System_Trigger."Load Configuration" ("System Trigger")) -> ()  [unwired: 12 in, 2 out]
      }
      event "Exit": Value Change {
        n180 = event-data() -> ()  [unwired: 2 out]
        n181 = call "EnQueue Trigger.vi"("trigger queue in"=w328, "system trigger"=System_Trigger."<Close Application>" ("System Trigger")) -> ()  [unwired: 12 in, 2 out]
      }
      event "Active Tab Selector": Value Change {
        n182 = event-data() -> ("NewVal"=w330:i32)  [unwired: 1 out]
        n183 = local write "Main Tab"(w330) -> ()
      }
      event "Main Tab": Value Change {
        n184 = event-data() -> ("NewVal"=w331:T1)  [unwired: 1 out]
        n185 = local write "Active Tab Selector"(w331) -> ()
      }
    }
  }
  n186 = Unbundle By Name(w4) -> ("Exit Event"=w3:refnum<user-event>)
  n187 = register-events(w3, w1) -> (reference out=w2:refnum<event-registration>)  [unwired: 2 in, 1 out]
  n188 = while {
    tunnel: w2 -> [w332]
    stop <- w333 stop-if-true
    n189 = event shown="[1] <Preferences Button>: Value Change" {
      selector: w332 -> [_ _]
      dyn-events: _ -> [_ _]
      timeout: _ -> [_ _]
      tunnel: [TRUE _] -> w333
      event User Event {
        n190 = event-data() -> ()  [unwired: 1 in, 3 out]
      }
      event Value Change {
        w344 = i16 623 ("y")
        w341 = i16 75 ("y")
        n191 = event-data() -> ("NewVal"=w345:bool)  [unwired: 1 in]
        n192 = control-ref of="Splitter 5"() -> (w335:refnum<vi>)
        n193 = control-ref of="Splitter 3"() -> (w336:refnum<vi>)
        n194 = property class="Splitter"(reference=w336) -> ("Position"=w348:i32, "Left"=w339:i32)  [unwired: 1 in, 2 out]
        n195 = property class="Splitter"(reference=w335) -> ("Position"=w343:i32)  [unwired: 1 in, 2 out]
        n196 = Negate(x=w341) -> (-x=w340:i16)
        n197 = Select(t=w341, s=w345, f=w340) -> (s? t:f=w342:i16)
        n198 = Add(x=w348, y=11) -> (x+y=w346:i32)
        n199 = Add(x=w339, y=10) -> (x+y=w337:i32)
        n200 = while {
          tunnel: w335 -> [w362]
          tunnel: w342 -> [w360]
          tunnel: w343 -> [w354]
          tunnel: [w351] -> w349
          tunnel: w344 -> [w350]
          i -> [w361]
          stop <- w358 stop-if-true
          n201 = Increment(x=w361) -> (x+1=w353:i32)
          n202 = Multiply(x=w360, y=w353) -> (x*y=w357:i32)
          n203 = Add(x=w354, y=w357) -> (x+y=w355:i32)
          n204 = Greater Or Equal?(x=w355, y=w350) -> (x >= y?=w356:bool)
          n205 = property class="Splitter"(reference=w362, "Position"=w355) -> (reference out=w351:refnum<vi>, error out=w359:errorcluster)  [unwired: 1 in]
          n206 = Or(x=w359, y=w356) -> (x .or. y?=w358:bool)
          n207 = Wait (ms)(milliseconds to wait=u32 25) -> ()  [unwired: 1 out]
        }
        n208 = case shown="False" w345 {
          tunnel: w349 -> [w364 w366]
          tunnel: w346 -> [w363 _]
          tunnel: w344 -> [_ w365]
          tunnel: w337 -> [_ _]
          frame False {
            n209 = property class="Splitter"(reference=w364, "Position"=w363) -> ()  [unwired: 1 in, 2 out]
          }
          frame True {
            n210 = property class="Splitter"(reference=w366, "Position"=w365) -> ()  [unwired: 1 in, 2 out]
          }
        }
      }
    }
  }
  n211 = while {
    shift-right: [w376] -> _
    shift-left: T3."Close Display" -> [w369]
    tunnel: w17 -> [w374]
    tunnel: w12 -> [w375]
    tunnel: [w372] -> w19
    shift-right: [w371] -> w8
    shift-left: w16 -> [w373]
    tunnel: w11 -> [w370]
    i -> [w367]
    stop <- w368 stop-if-true
    # "Application Close"
    n212 = case shown="\"Clear References\"" w369 {
      tunnel: [w379 w389 w394] -> w372
      tunnel: [w378 w388 w391] -> w371
      tunnel: [w380 _ w393] -> _
      tunnel: w375 -> [w379 w389 w394]
      tunnel: w374 -> [w380 w387 w393]
      tunnel: w373 -> [w378 w388 w391]
      tunnel: w370 -> [w377 w385 w392]
      tunnel: [w377 _ w392] -> _
      frame "Close Display" {
        n213 = disable-structure shown="RUN_TIME_ENGINE==True" {
          disable-tunnel: w378 -> [_ w382]
          frame condition #0 (active) {
          }
          frame condition #1 {
            n214 = Unbundle By Name(w382) -> ("MAIN VI Refnum"=w381:refnum<vi>)
            n215 = invoke class="VI" method="FP.Open"(reference=w381, "Activate"=TRUE ("Activate?"), "State"=T9."Hidden") -> ()  [unwired: 2 in, 5 out]
          }
        }
      }
      frame "Clear References" {
        n216 = Unregister For Events(event registration refnum=w385) -> ()  [unwired: 1 in, 1 out]
        n217 = Unbundle By Name(w388) -> ("Framework Events"=w386:T7)
        n218 = Unregister For Events(event registration refnum=w387) -> ()  [unwired: 1 in, 1 out]
        n219 = call "Destroy CORE UI Display Events.vi"("UI display events in"=w386) -> ()  [unwired: 14 in, 1 out]
      }
      frame "Close Error Handler" {
        n220 = Unbundle By Name(w391) -> ("Error Handler"=w390:refnum<class "TLB` Error Handler.lvclass">)
        n221 = call-dynamic "Close.vi"("error handler in"=w390) -> ()  [unwired: 14 in, 1 out]
      }
    }
    n222 = call "Enum Loop Complete.vi"("Current State Enum"=w369, "Itteration"=w367) -> ("Loop Complete?"=w368:bool)  [unwired: 12 in, 1 out]
    n223 = Increment(x=w369) -> (x+1=w376:T3)
  }
  n224 = disable-structure shown="RUN_TIME_ENGINE==True" {
    disable-tunnel: [w395 w396] -> w6
    disable-tunnel: w19 -> [w395 w397]
    frame condition #0 (active) {
    }
    frame condition #1 {
      n225 = flat-sequence {
        tunnel: [w398] -> w396
        tunnel: w397 -> [w398]
        frame #0 {
          n226 = Quit LabVIEW() -> ()  [unwired: 1 in]
        }
      }
    }
  }
  n227 = Unbundle By Name(w8) -> ("Terminate Error"=w7:errorcluster)
  n228 = Merge Errors(w7, w6) -> (→"error out":errorcluster)
